vi "Power scan Track and SPCM.vi"() -> ()   [LabVIEW 2012]
uses:
  F:/Users/Ouyang Group/Documents/Colton LabView code/Instruments/Laser power controller/BEOC LPC/BEOC LPC.lvlib
panel:
  out "Power":dbl
  in  "Z interval (min)":dbl
  out "Z Position 2":dbl
  out "Y Position":dbl
  out "X Position":dbl
  in  "Data File Path":path=path "C:/Users/Ouyang Group/Documents/Calibration pictures/Nanodiamond/8-5-13/X=192 Y=35 1mW 800 sp filter 4 hours position tracking.txt"
  in  "Scan Interval (minutes)":dbl=7.0
  in  "Collection Time (hours)":dbl=4.0
  in  "Z Position":dbl=52.1
  in  "Y pos":dbl=35.0
  in  "X Pos":dbl=192.0
  in  "Y Parameters":T1={"Number of Y Steps"=200, "Max Y (V)"=2.0, "Min Y (V)"=-2.0}
  in  "X Parameters":T2={"Number of X Steps"=200, "Max X (V)"=2.0, "Min X (V)"=-2.0}
  in  "RS232 settings":cluster{"Portnumber":i32, "Baudrate":u16}={"Portnumber"=12, "Baudrate"=5} {"Portnumber" items=["COM1", "COM2", "COM3", "COM4", "COM5", "COM6", "COM7", "COM8", "COM9", "COM10", "COM11", "COM12", "COM13", "COM14", "COM15", "COM16", "COM17", "COM18", "COM19", "COM20", "COM21", "COM22", "COM23", "COM24", "COM25", "COM26", "COM27", "COM28", "COM29", "COM30"]; "Baudrate" items=["9600", "14400", "19200", "38400", "57600", "115200"]}
  out "LPC found?":bool
  in  "Array - Numeric":dbl[](array[numeric])
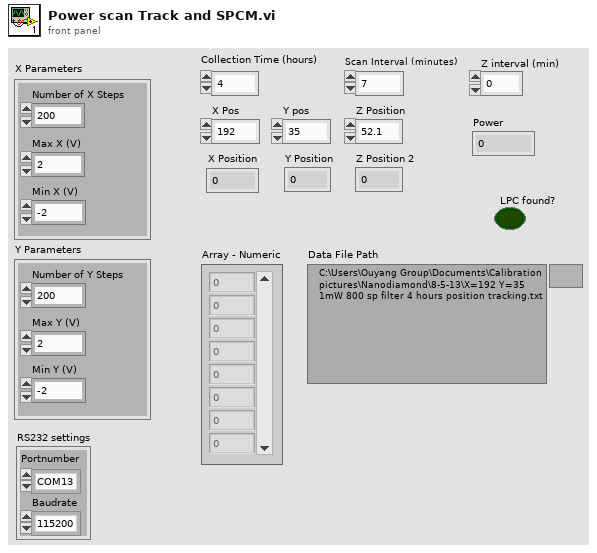
[diagram p1: front panel]
types:
  T1 = cluster{"Number of Y Steps":i32, "Max Y (V)":dbl, "Min Y (V)":dbl}
  T2 = cluster{"Number of X Steps":i32, "Max X (V)":dbl, "Min X (V)":dbl}
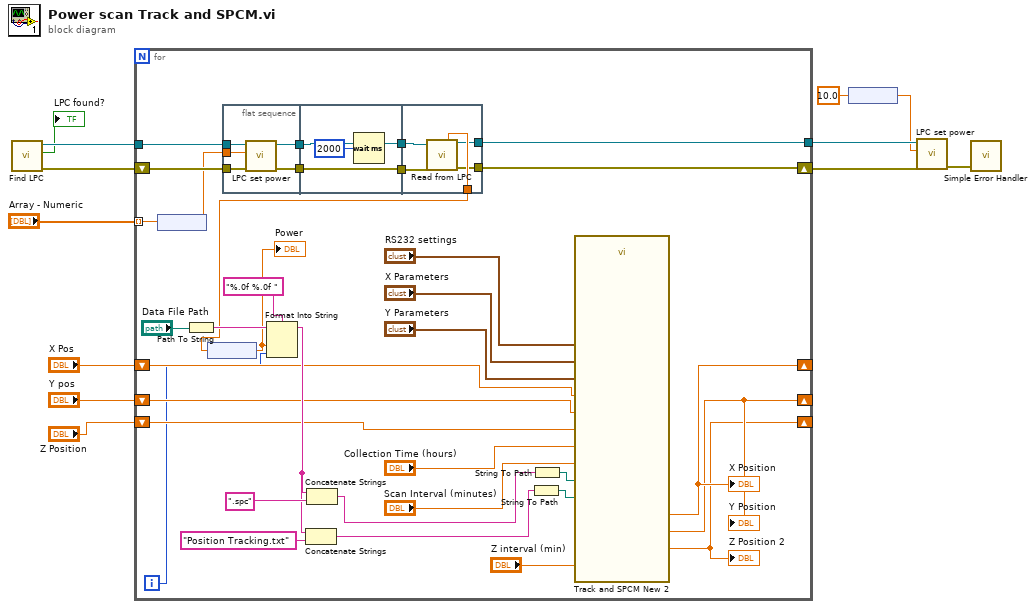
[diagram p0: block diagram]
diagram:
  n1 = call "Find LPC.vi"() -> ("error out"=w10:errorcluster, "LPC found?"=→"LPC found?":bool, "VISA resource name out"=w11:refnum<visa-resource-name>)  [unwired: 2 in, 7 out]
  n2 = for {
    tunnel: "Array - Numeric" -> [w45] mode=indexing
    tunnel: w11 -> [w47]
    shift-right: [w39] -> w4
    shift-left: w10 -> [w46]
    shift-right: [w23] -> _
    shift-left: "X Pos" -> [w26]
    shift-right: [w22] -> _
    shift-left: "Y pos" -> [w25]
    shift-right: [w21] -> _
    shift-left: "Z Position" -> [w24]
    tunnel: [w17] -> w5
    i -> [w16]
    n3 = node(w45) -> (w44:dbl[unit])
    n4 = Path To String(path="Data File Path") -> (string=w32:string)
    n5 = node(w19) -> (w18:dbl)
    "Power" <- w18
    n6 = flat-sequence {
      tunnel: w47 -> [w52]
      tunnel: w46 -> [w51]
      tunnel: w44 -> [w50]
      tunnel: [w49] -> w43
      tunnel: [w48] -> w42
      tunnel: w43 -> [w54]
      tunnel: w42 -> [w53]
      tunnel: [w54] -> w41
      tunnel: [w53] -> w40
      tunnel: w41 -> [w60]
      tunnel: w40 -> [w59]
      tunnel: [w58] -> w19
      tunnel: [w57] -> w39
      tunnel: [w56] -> w17
      frame #0 {
        n7 = call "LPC set power.vi"("error in (no error)"=w51, "power"=w50, "VISA resource name"=w52) -> ("error out"=w48:errorcluster, "VISA resource name out"=w49:refnum<visa-resource-name>)  [unwired: 7 in]
      }
      frame #1 {
        n8 = Wait (ms)(milliseconds to wait=u32 2000) -> ()  [unwired: 1 out]
      }
      frame #2 {
        n9 = call "Read from LPC.vi"("VISA resource name"=w60, "error in (no error)"=w59) -> ("power"=w58:dbl[unit], "VISA resource name out"=w56:refnum<visa-resource-name>, "error out"=w57:errorcluster)  [unwired: 7 in, 4 out]
      }
    }
    n10 = Format Into String(format string="%.0f %.0f ", initial string=w32, w18, w16) -> (resulting string=w27:string)  [unwired: 1 in, 1 out]
    n11 = Concatenate Strings(w27, "Position Tracking.txt" ("string")) -> (w28:string)
    n12 = Concatenate Strings(w27, ".spc" ("string")) -> (w29:string)
    n13 = String To Path(string=w28) -> (path=w13:path)
    n14 = String To Path(string=w29) -> (path=w14:path)
    n15 = call "Track and SPCM New 2.vi"("X Parameters"="X Parameters", "X Pos"=w26, "Scan Interval (minutes)"="Scan Interval (minutes)", "Y pos"=w25, "Y Parameters"="Y Parameters", "Z interval (min)"="Z interval (min)", "RS232 settings"="RS232 settings", "Z Pos"=w24, "SPCM File Path"=w14, "Collection Time (hours)"="Collection Time (hours)", "Tracking Data File Path"=w13) -> ("X Position"=w23:dbl, "Y Position"=w22:dbl, "Z Position"=w21:dbl)  [unwired: 2 in]
    "X Position" <- w23
    "Y Position" <- w22
    "Z Position 2" <- w21
  }
  n16 = node(10.0) -> (w2:dbl[unit])
  n17 = call "LPC set power.vi"("error in (no error)"=w4, "power"=w2, "VISA resource name"=w5) -> ("error out"=w1:errorcluster)  [unwired: 7 in, 1 out]
  n18 = call <vilib>:"Simple Error Handler.vi"("error in (no error)"=w1) -> ()  [unwired: 4 in, 5 out]
